vi "Create.vi"(10 "Channel":refnum<class "Channel BOOL.lvclass">) -> (3 "BoolChannelValue out":refnum<class "BoolChannelValue.lvclass">)   [LabVIEW 2020, in "Vecto.lvlib" / "BoolChannelValue.lvclass"]
uses:
  BoolChannelValue.lvclass
  BoolChannelValue.lvclass/BoolChannelValue.ctl
  Channel BOOL/Channel BOOL.lvclass
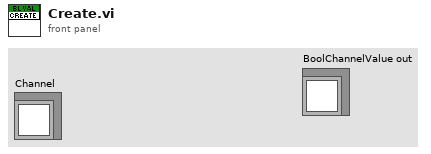
[diagram p1: front panel]
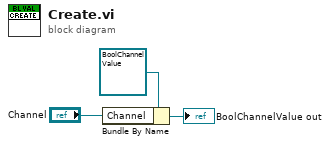
[diagram p0: block diagram]
diagram:
  n1 = Bundle By Name(cluster=refnum<class "BoolChannelValue.lvclass"> refnum ("BoolChannelValue in"), "Channel"="Channel") -> (→"BoolChannelValue out":refnum<class "BoolChannelValue.lvclass">)
